vi "Use.vi"(8 "error in (no error)":errorcluster, 10 "Configuration ID":string, 11 "CLI Client in":refnum<class "JFrog CLI.lvclass">) -> (0 "error out":errorcluster, 1 "Ellapsed Time [Sec]":dbl, 3 "CLI Client out":refnum<class "JFrog CLI.lvclass">)   [LabVIEW 2015, in "JFrog CLI.lvclass"]
uses:
  JFrog CLI.lvclass
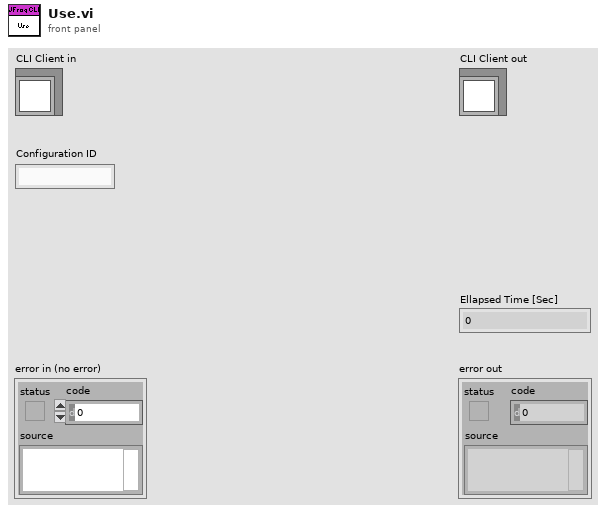
[diagram p1: front panel]
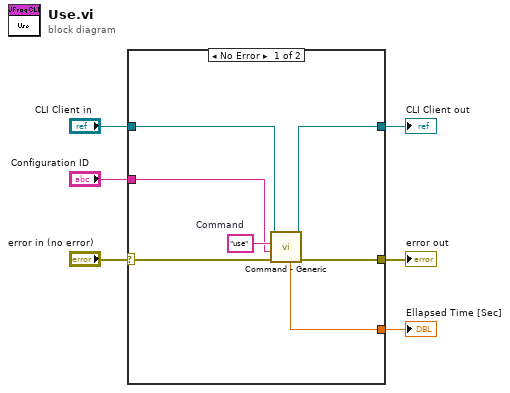
[diagram p0: block diagram]
diagram:
  n1 = case shown="No Error" "error in (no error)" {
    selector: "error in (no error)" -> [w13 w15]
    tunnel: [w12 w15] -> w4
    tunnel: [w10 w14] -> w3
    tunnel: "CLI Client in" -> [w11 w14]
    tunnel: "Configuration ID" -> [w8 _]
    tunnel: [w7 _] -> w1
    frame No Error {
      w9 = "use"  # Command
      n2 = call "Command - Generic.vi"("error in (no error)"=w13, "Parameters"=w8, "Command"=w9, "CLI Client in"=w11) -> ("error out"=w12:errorcluster, "CLI Client out"=w10:refnum<class "JFrog CLI.lvclass">, "Ellapsed Time [Sec]"=w7:dbl)  [unwired: 3 in, 2 out]
    }
    frame Error {
    }
  }
  "error out" <- w4
  "CLI Client out" <- w3
  "Ellapsed Time [Sec]" <- w1
